vi "AES-Cipher-BLOCK.vi"(8 "error in (no error)":errorcluster, 10 "Cipher Key":u8[](array[numeric]) format="%02x", 11 "Plain [U8]":u8[](array[numeric]) format="%02x") -> (0 "error out":errorcluster, 3 "cipher [U8]":u8[](array[numeric]) format="%02x")   [LabVIEW 2020, in "Encryption.lvlib"]
doc: "Encripts the U8 block (16 bytes) using AES with the given cipher.\n\nCAUTION:\nThis VI is not secure, it does not protect the memory of the encryption, key and unencrypted data.\n\n(c) Ton Plomp, 2011\nTHIS SOFTWARE IS PROVIDED AS IS, AND ANY WARRANTY IS REJECTED"
uses:
  Encryption.lvlib
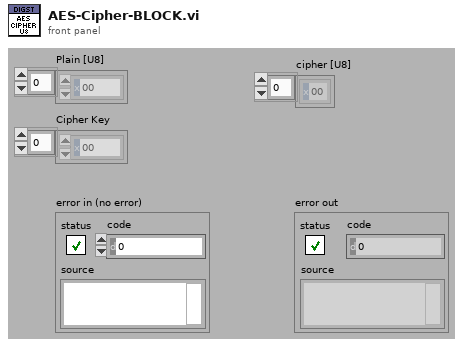
[diagram p1: front panel]
types:
  T1 = cluster{bool, i32, "String to Prepend to source (\"\")":string}
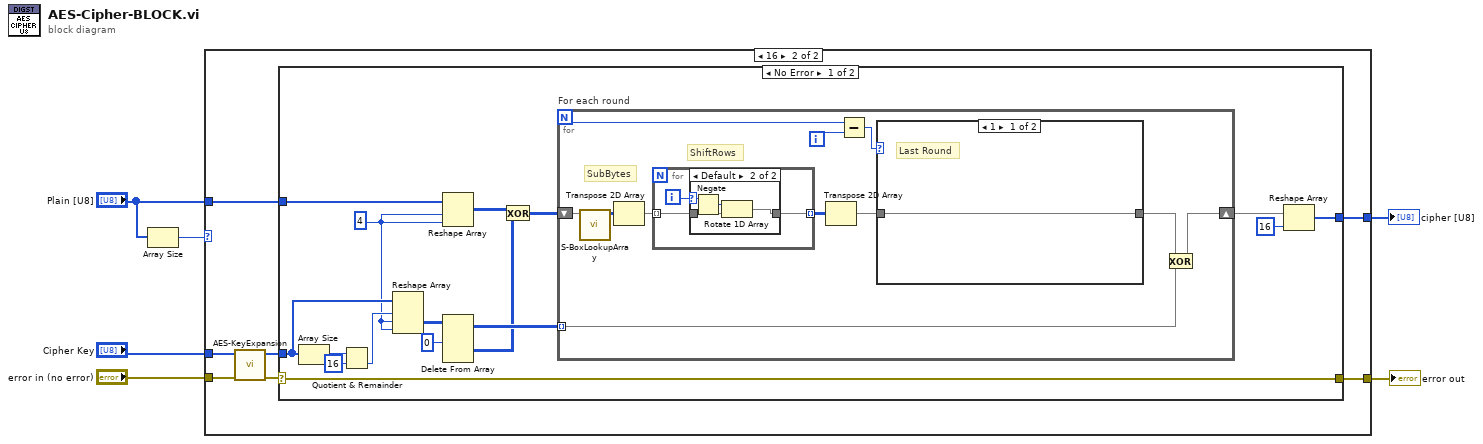
[diagram p0: block diagram]
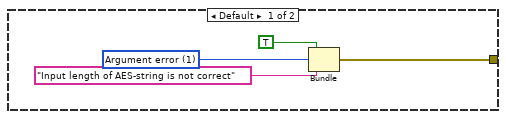
[diagram p2: hidden frame]
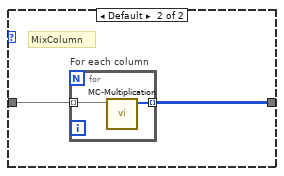
[diagram p3: hidden frame]
diagram:
  n1 = Array Size(array="Plain [U8]") -> (size(s)=w2:i32)
  n2 = case shown="16" w2 {
    tunnel: [_ w16] -> w6
    tunnel: "Cipher Key" -> [_ w15]
    tunnel: "error in (no error)" -> [_ w14]
    tunnel: "Plain [U8]" -> [_ w13]
    tunnel: [w7 w11] -> w1
    frame Default {
      w8 = 1 items=["No error", "Argument error", "Memory is full", "Out of zone", "End of file", "File already open", "Generic file I/O error", "File not found", "File permission error", "Disk is full", "Duplicate path", "Too many files open", "System feature not enabled", "Resource file not found", "Cannot add resource", "Resource not found", "Image not found", "Image memory error", "Pen does not exist", "Config type invalid", "Config token not found", "Config parse error", "Config memory error", "Bad external code format", "Bad external code offset", "External code not present", "Null window", "Destroy window error", "Null menu", "Print aborted", "Bad print record", "Print driver error", "Windows error during printing", "Memory error during printing", "Print dialog error", "Generic print error", "Invalid device refnum", "Device not found", "Device parameter error", "Device unit error", "Cannot open device", "Device call aborted", "Generic error", "Cancelled by user", "Object ID too low", "Object ID too high", "Object not in heap", "Unknown heap", "Unknown object (invalid DefProc)", "Unknown object (DefProc not in table)", "Message out of range", "Invalid (null) method", "Unknown message", "Manager call not supported", "Bad address", "Network operation in progress", "Network operation timed out", "Connection is busy", "Network attribute not supported", "Network error", "Address in use", "System out of memory", "Connection aborted", "Connection refused", "Not connected", "Already connected", "Connection closed", "Initialization error (interapplication manager)", "Bad occurrence", "Wait on unbound occurrence handler", "Occurrence queue overflow", "Datalog type conflict", "Unused", "Unrecognized type (interapplication manager)", "Memory corrupt", "Failed to make temporary DLL", "Old CIN version", "Drag socket not found", "Failed to load drop-object", "Failed to register OLE object", "Failed to release OLE object", "Format specifier type mismatch", "Unknown format specifier", "Too few format specifiers", "Too many format specifiers", "Scan failed", "Newer CIN version", "Error converting to variant", "Runtime menu error", "Password tampered", "Variant attribute not found", "Incompatible variant data type", "Event data is not available", "Event Store is not present", "Occurrence is not found", "Event Queue is not created", "Event info is not available", "Refnum passed is NULL", "Error retrieving Class GUID", "Error retrieving CoClass GUID", "Error retrieving TypeLib GUID.", "Bad built application magic bytes.", "Specific driver is different from the specific driver associated with the Logical Name.", "There is no session opened to the class driver.", "Max Error", "MAX - Error with config objects", "MAX - Error loading configuration", "MAX - Group not supported"]
      n3 = Bundle(TRUE, w8, "String to Prepend to source (\"\")"="Input length of AES-string is not correct" ("String to Prepend to source (\"\")")) -> (w7:T1)  [unwired: 1 in]
    }
    frame 16 {
      n4 = call "AES-KeyExpansion.vi"("error in (no error)"=w14, "Key In"=w15) -> ("error out"=w12:errorcluster, "Expanded Key [U8]"=w17:u8[])  [unwired: 8 in]
      n5 = case shown="No Error" w12 {
        selector: w12 -> [w21 w58]
        tunnel: w17 -> [w31 _]
        tunnel: [w25 _] -> w16
        tunnel: w13 -> [w23 _]
        tunnel: [w21 w58] -> w11
        frame No Error {
          w22 = 4 ("y")
          n6 = Array Size(array=w31) -> (size(s)=w33:i32)
          n7 = Quotient & Remainder(x=w33, y=16) -> (floor(x/y)=w28:i32)  [unwired: 1 out]
          n8 = Reshape Array(w31, w28, w22, w22) -> (w18:u8[][][])
          n9 = Reshape Array(w23, w22, w22) -> (w20:u8[][])
          n10 = Delete From Array(array=w18, index (dim 0)=0 ("disabled index (col)")) -> (deleted portion=w19:u8[][], array with subset deleted=w30:u8[][][])  [unwired: 3 in]
          n11 = Exclusive Or(1:w19, 2:w20) -> (0:w29:u8[][])
          n12 = for "For each round" {
            N -> [w42]
            shift-right: [w38] -> w26
            shift-left: w29 -> [w44]
            tunnel: w30 -> [w39] mode=indexing
            i -> [w41]
            # "ShiftRows"
            # "SubBytes"
            n13 = call "S-BoxLookupArray.vi"("In"=w44) -> ("Out"=w37:u8[][])  [unwired: 10 in]
            n14 = Transpose 2D Array(2D array=w37) -> (transposed array=w35:u8[][])
            n15 = for {
              tunnel: w35 -> [w51] mode=indexing
              tunnel: [w50] -> w36 mode=indexing
              i -> [w52]
              n16 = case shown="Default" w52 {
                selector: w52 -> [_ w56]
                tunnel: w51 -> [w53 w57]
                tunnel: [w53 w55] -> w50
                frame 0 {
                }
                frame Default {
                  n17 = Negate(x=w56) -> (-x=w54:i32)
                  n18 = Rotate 1D Array(1:w57, 2:w54) -> (0:w55:u8[])
                }
              }
            }
            n19 = Transpose 2D Array(2D array=w36) -> (transposed array=w34:u8[][])
            n20 = Subtract(x=w42, y=w41) -> (x-y=w40:i32)
            n21 = case shown="1" w40 {
              tunnel: w34 -> [w45 w47]
              tunnel: [w45 w46] -> w43
              frame 1 {
                # "Last Round"
              }
              frame Default {
                # "MixColumn"
                n22 = for "For each column" {
                  tunnel: w47 -> [w48] mode=indexing
                  tunnel: [w49] -> w46 mode=indexing
                  n23 = call "MC-Multiplication.vi"("Vector In"=w48) -> ("Vector Out"=w49:u8[])  [unwired: 10 in]
                }
              }
            }
            n24 = Exclusive Or(1:w39, 2:w43) -> (0:w38:u8[][])
          }
          n25 = Reshape Array(w26, 16 ("dimension size")) -> (w25:u8[])
        }
        frame Error {
        }
      }
    }
  }
  "error out" <- w1
  "cipher [U8]" <- w6
